vi "Start DAQ.vi"(8 "error in (no error)":errorcluster, 11 "TDMS DAQ in":refnum<class "TDMS DAQ.lvclass">) -> (0 "error out":errorcluster, 3 "TDMS DAQ out":refnum<class "TDMS DAQ.lvclass">)   [LabVIEW 2025, in "TDMS DAQ.lvlib" / "TDMS DAQ.lvclass"]
uses:
  TDMS DAQ.lvclass
  TDMS DAQ.lvclass/TDMS DAQ.ctl
  DAQ Interface/DAQ Interface/DAQ Interface.lvclass
  Helper Loop Type.ctl
  Helper Loop Message.ctl
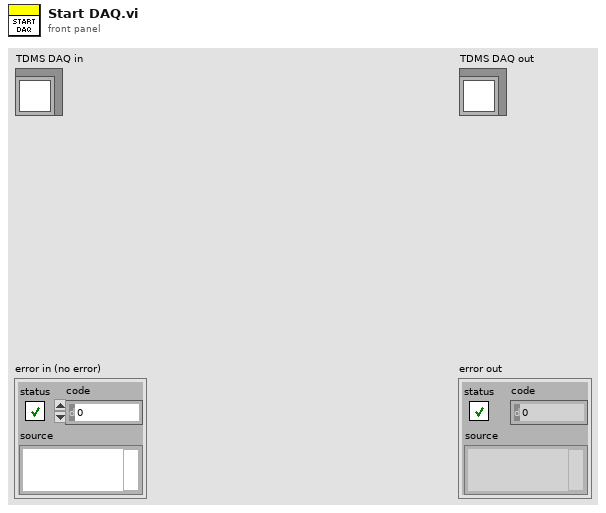
[diagram p1: front panel]
types:
  T1 = typedef "TDMS DAQ.lvlib/TDMS DAQ.lvclass/Helper Loop Message.ctl" = cluster{"Type":T2, "Payload":variant}
  T2 = typedef "TDMS DAQ.lvlib/TDMS DAQ.lvclass/Helper Loop Type.ctl" = enum16{"Configure", "Start", "Do", "Stop", "Clean", "Close"}
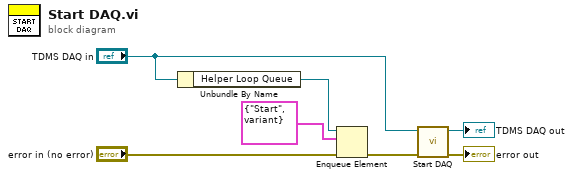
[diagram p0: block diagram]
diagram:
  n1 = Unbundle By Name("TDMS DAQ in") -> ("Helper Loop Queue"=w4:refnum<queue>)
  n2 = Enqueue Element(queue=w4, element=T1 {"Type"=enum."Start", "Payload"=variant}, error in (no error)="error in (no error)") -> (error out=w2:errorcluster)  [unwired: 1 in, 2 out]
  n3 = call-parent "Start DAQ.vi"("error in (no error)"=w2, "DAQ Interface in"="TDMS DAQ in") -> ("error out"=→"error out":errorcluster, "DAQ Interface out"=→"TDMS DAQ out":refnum<class "TDMS DAQ.lvclass">)  [unwired: 8 in]
